vi "CloseConnectionToIrDAServer.vi"(3 "IrDA Refnum":refnum<k19>) -> (0 "error out":errorcluster)   [LabVIEW 2013]
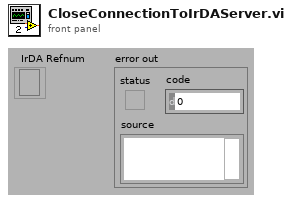
[diagram p1: front panel]
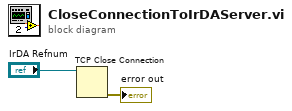
[diagram p0: block diagram]
diagram:
  n1 = TCP Close Connection(connection ID="IrDA Refnum") -> (error out=→"error out":errorcluster)  [unwired: 1 in, 2 out]
